vi "eng-call-start.vi"(8 "error in (no error)":errorcluster, 10 "Start(T)/Stop(F)":bool) -> (0 "error out":errorcluster)   [LabVIEW 2024]
uses:
  controls/state-engine.ctl
  globals/globals-engine.vi
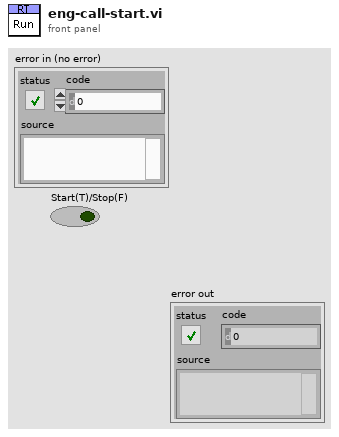
[diagram p1: front panel]
types:
  T1 = typedef "state-engine.ctl" = enum16{"ENG.NO-OP", "ENG.START", "ENG.STOP", "ENG.EXECUTE", "ENG.STATUS", "ENG.EXTERNAL-CALL", "ENG.INIT", "ENG.INIT.VARS", "ENG.INIT.SERIAL", "ENG.LOAD", "ENG.LOAD.SINGLE", "ENG.LOAD.MODULE", "ENG.LOAD.RELOAD", "ENG.LOAD.UNLOAD", "ENG.IO.LOAD", "ENG.IO.SAVE", "ENG.PROC.RELOAD-BY-NAME", "ENG.PROC.START", "ENG.PROC.STOP", "ENG.PROC.INSERT-STEPS", "ENG.PROC.ISRUNNING", "ENG.PROC.PRESET", "ENG.PROC.STATUS", "ENG.PRINT-USER-MSG", "ENG.RIO.SNAPSHOT", "ENG.RIO.AIN-SNAPSHOT-CALIB", "ENG.RIO.DOUT-BY-ADDR", "ENG.RIO.DOUT-BY-NAME", "ENG.RIO.RFS-DELAY-SET-X1", "ENG.RIO.RFS-DELAY-SET-X8", "ENG.RIO.RFS-CYCLES-SET", "ENG.RIO.RFS-CYCLES-GET", "ENG.RIO.RFS-ENABLE", "ENG.EXIT"}
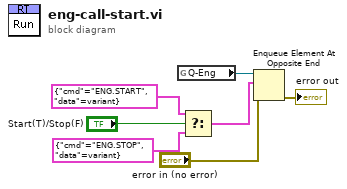
[diagram p0: block diagram]
diagram:
  n1 = global read "globals-engine.vi" "Q-Eng"() -> (w6:refnum<queue>)
  n2 = Select(t=cluster{"cmd":T1, "data":variant} {"cmd"=enum."ENG.START", "data"=variant} ("typedefElement"), s="Start(T)/Stop(F)", f=cluster{"cmd":T1, "data":variant} {"cmd"=enum."ENG.STOP", "data"=variant} ("typedefElement")) -> (s? t:f=w2:cluster{"cmd":T1, "data":variant})
  n3 = Enqueue Element At Opposite End(queue=w6, element=w2, error in (no error)="error in (no error)") -> (error out=→"error out":errorcluster)  [unwired: 1 in, 2 out]
